vi "2D to 1D.vi"(11 "DetailTestResult":string[][](array[string])) -> (2 "data":string[](array[string]), 3 "head":string[](array[string]))   [LabVIEW 2025, in "Test Unit.lvlib"]
uses:
  Test Unit.lvlib
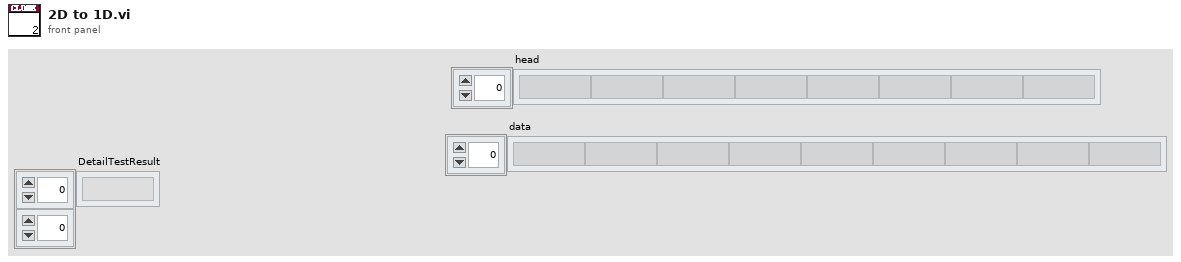
[diagram p1: front panel]
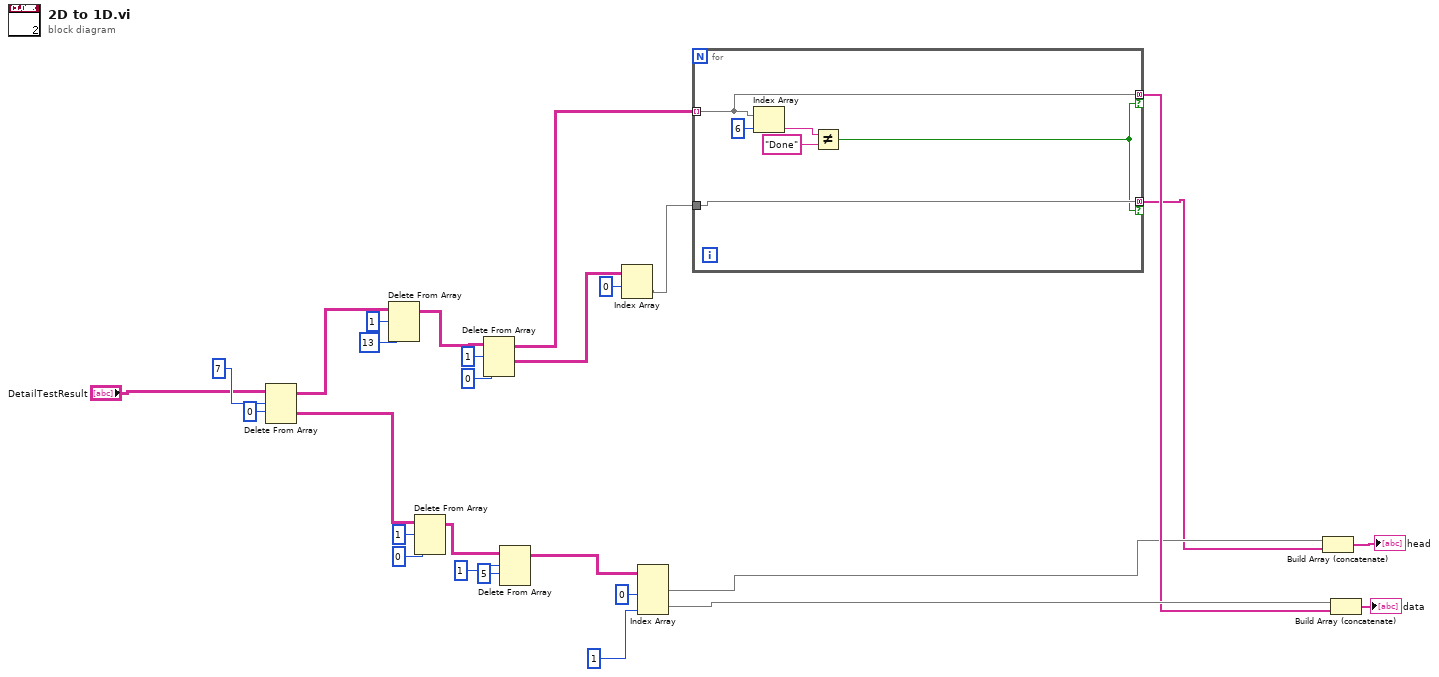
[diagram p0: block diagram]
diagram:
  n1 = Delete From Array(array="DetailTestResult", length=7, index (row)=0) -> (deleted portion=w26:string[][], array with subset deleted=w4:string[][])  [unwired: 1 in]
  n2 = Delete From Array(array=w4, length=1, index (col)=13 ("disabled index (col)")) -> (array with subset deleted=w1:string[][])  [unwired: 1 in, 1 out]
  n3 = Delete From Array(array=w26, length=1, index (row)=0) -> (array with subset deleted=w23:string[][])  [unwired: 1 in, 1 out]
  n4 = Delete From Array(array=w1, length=1, index (row)=0) -> (deleted portion=w14:string[][], array with subset deleted=w15:string[][])  [unwired: 1 in]
  n5 = Delete From Array(array=w23, length=1, index (row)=5) -> (array with subset deleted=w20:string[][])  [unwired: 1 in, 1 out]
  n6 = Index Array(array=w14, index (row)=0) -> (element=w12:string[])  [unwired: 1 in]
  n7 = Index Array(array=w20, index (col) #1=0 ("disabled index (col)"), index (col) #2=1 ("index (col)")) -> (element #1=w8:string[], element #2=w11:string[])  [unwired: 2 in]
  n8 = for {
    tunnel: w15 -> [w31] mode=indexing
    tunnel: [w31] -> w10 mode=concatenating if=w29
    tunnel: w12 -> [w30]
    tunnel: [w30] -> w7 mode=concatenating if=w29
    n9 = Index Array(array=w31, index=6) -> (element=w33:string)
    n10 = Not Equal?(x=w33, y="Done") -> (x != y?=w29:bool)
  }
  n11 = Build Array (concatenate)(w8, w7) -> (→"head":string[])
  n12 = Build Array (concatenate)(w11, w10) -> (→"data":string[])
